vi "Set_LEDs.vi"(11 "RelayValue":T5) -> (3 "RelayDevRef":T1={"DevStatus"={"status"=FALSE, "code"=0, "source"=""}, "Relay Channel"=enum."Invalid", "Digital Module"=enum."Digital Module 1", "Relay Direction"=enum."Both directions"})   [LabVIEW 2012]
uses:
  <vilib>/Rock Robotics/WPI/Relay/WPI_RelayValue.ctl
  <vilib>/Rock Robotics/WPI/Relay/WPI_RelayDevRef.ctl
  <vilib>/Rock Robotics/SystemInterfaces/DIO/FPGA_DIORelayChannel.ctl
  <vilib>/Rock Robotics/SystemInterfaces/Typedef/FPGA_TypedefDigitalModule.ctl
  <vilib>/Rock Robotics/WPI/Relay/WPI_RelayDirection.ctl
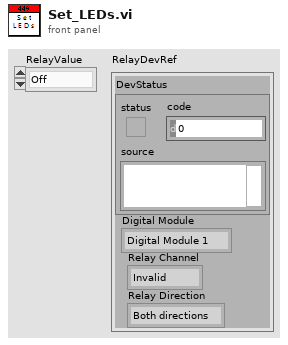
[diagram p1: front panel]
types:
  T1 = typedef "WPI_RelayDevRef.ctl" = cluster{"DevStatus":errorcluster, "Relay Channel":T2, "Digital Module":T3, "Relay Direction":T4}
  T2 = typedef "FPGA_DIORelayChannel.ctl" = enum8{"Relay 1", "Relay 2", "Relay 3", "Relay 4", "Relay 5", "Relay 6", "Relay 7", "Relay 8", "Invalid"}
  T3 = typedef "FPGA_TypedefDigitalModule.ctl" = enum16{"Digital Module 1", "Digital Module 2"}
  T4 = typedef "WPI_RelayDirection.ctl" = enum16{"Both directions", "Forward only", "Reverse only"}
  T5 = typedef "WPI_RelayValue.ctl" = enum16{"Off", "On", "Forward", "Reverse"}
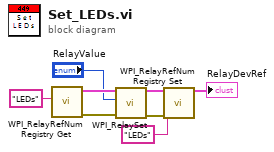
[diagram p0: block diagram]
diagram:
  n1 = call <vilib>:"WPI_RelayRefNum Registry Get.vi"("refnum name"="LEDs") -> ("error out"=w7:errorcluster, "RelayDevRef"=w6:T1)  [unwired: 9 in]
  n2 = call <vilib>:"WPI_RelaySet.vi"("error in (no error)"=w7, "RelayValue"="RelayValue", "RelayDevRef"=w6) -> ("error out"=w1:errorcluster, "RelayDevRef"=w4:T1)  [unwired: 7 in]
  n3 = call <vilib>:"WPI_RelayRefNum Registry Set.vi"("error in (no error)"=w1, "refnum name"="LEDs", "RelayDevRef"=w4) -> ("RelayDevRef"=→"RelayDevRef":T1)  [unwired: 7 in, 1 out]
